vi "Reset Dev.vi"(11 "devId":i32) -> (2 "devId out":i32, 3 "function return":i32)   [LabVIEW 2013, in "CHR34XXX.lvlib"]
doc: "DLL BOOL __stdcall CHR34XXX_OpenDev(IN int devId); DLL BOOL __stdcall CHR34XXX_OpenDevEx(OUT int *devId,IN BYTE busNo,IN BYTE DevNo,IN BYTE FuncNo); DLL BOOL __stdcall CHR34XXX_CloseDev(IN int devId); DLL BOOL __stdcall CHR34XXX_ResetDev(IN int devId);"
uses:
  CHR34XXX.lvlib
  CHR34XXX.dll
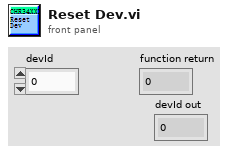
[diagram p1: front panel]
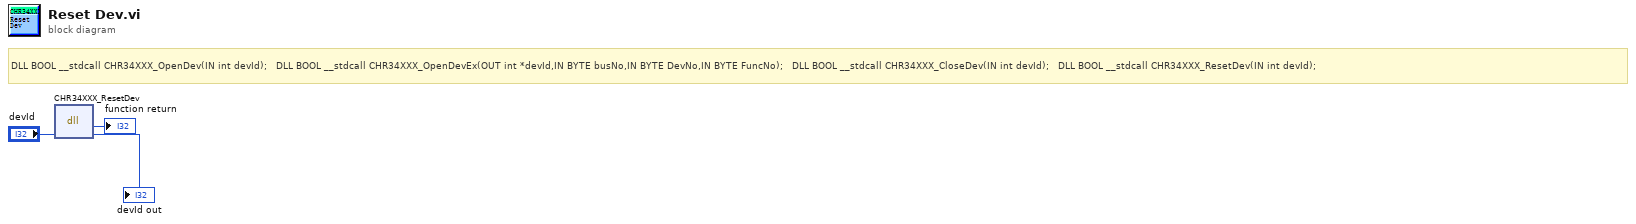
[diagram p0: block diagram]
diagram:
  # "DLL BOOL __stdcall CHR34XXX_OpenDev(IN int devId);   DLL BOOL __stdcall CHR34XXX_OpenDevEx(OUT int *devId,IN BYTE busNo,IN BYTE DevNo,IN BYTE FuncNo);   DLL BOOL __stdcall CHR34XXX_CloseDev(IN int devId);   DLL BOOL __stdcall CHR34XXX_ResetDev(IN int devId);"
  n1 = dll-call lib="C:/Users/dy/Desktop/CHR34XXX_lv/lv_lib/CHR34XXX.*" fn="CHR34XXX_ResetDev"("devId"="devId") -> ("返回类型"=→"function return":i32, "devId"=→"devId out":i32)  [unwired: 3 in, 2 out]
